vi "Timing Page.vi"(8 "error in (no error)":errorcluster, 11 "Node Ptr":T1 format="%.0x") -> (0 "error out":errorcluster)   [LabVIEW 2020, in "Engine Simulation Toolkit System Explorer.lvlib"]
uses:
  Engine Simulation Toolkit System Explorer.lvlib
  <vilib>/NI VeriStand/Custom Device API/Custom Device Item Ref.ctl
  Shared/Properties.vi
  <vilib>/NI VeriStand/Custom Device API/Get Item Property (Double).vi
  Shared/Constants and GUIDs.vi
  <vilib>/NI VeriStand/Custom Device API/Set Item Property (Double).vi
  <vilib>/NI VeriStand/Custom Device API/Custom Device API.lvlib
  Shared/Engine Simulation Toolkit Shared.lvlib
panel:
  in  "Stuck active\nlimit (ms)":dbl min=0.0 max=209.7152 step=0.0008
  in  "Header 2":cluster{"Section Name":string}={"Section Name"="Measurements"}
  in  "remove meas":bool
  in  "add meas":bool
  in  "remove windows":bool
  in  "add window":bool
  in  "windows listbox":i32[](listbox) caption="Window Definitions"
  in  "meas listbox":i32[](listbox) caption="Measurements"
  in  "Header":cluster{"Section Name":string}={"Section Name"="Measurement Windows"}
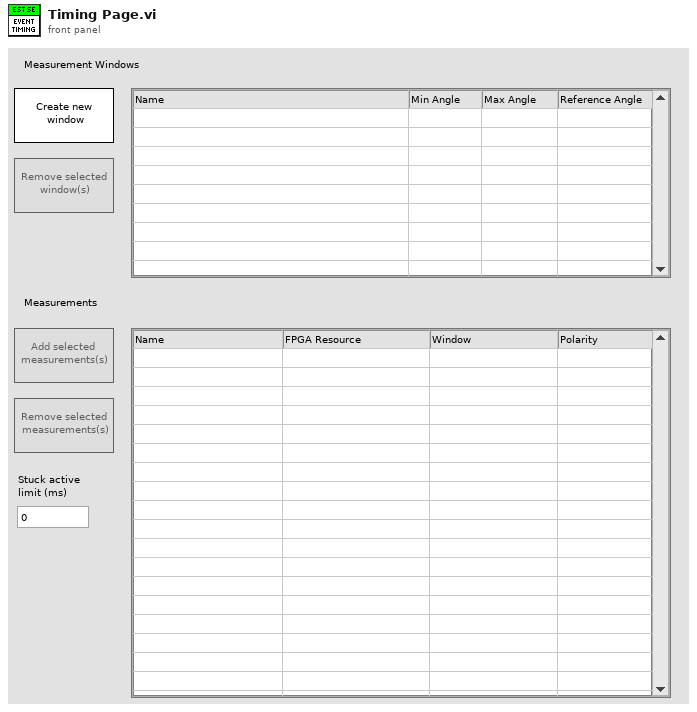
[diagram p1: front panel]
types:
  T1 = typedef "Custom Device API.lvlib/Custom Device Item Ref.ctl" = u64
  T2 = enum8{"Enabled", "Disabled", "Disabled and Grayed Out"}
  T3 = typedef "Engine Simulation Toolkit System Explorer.lvlib/Event Timing Window.ctl" = cluster{"Name":string, "Min":dbl, "Max":dbl, "Ref":dbl}
  T4 = typedef "Engine Simulation Toolkit System Explorer.lvlib/Event Timing Measurement.ctl" = cluster{"Name":string, "Bitfile name":string, "Window":string, "Polarity":T5}
  T5 = typedef "Engine Simulation Toolkit System Explorer.lvlib/Polarity.ctl" = enum16{"Active low", "Active high"}
  T6 = typedef "Custom Device API.lvlib/Custom Device Commands.ctl" = enum16{"Default", "Item renamed", "Shutdown", "Dynamic button pressed"}
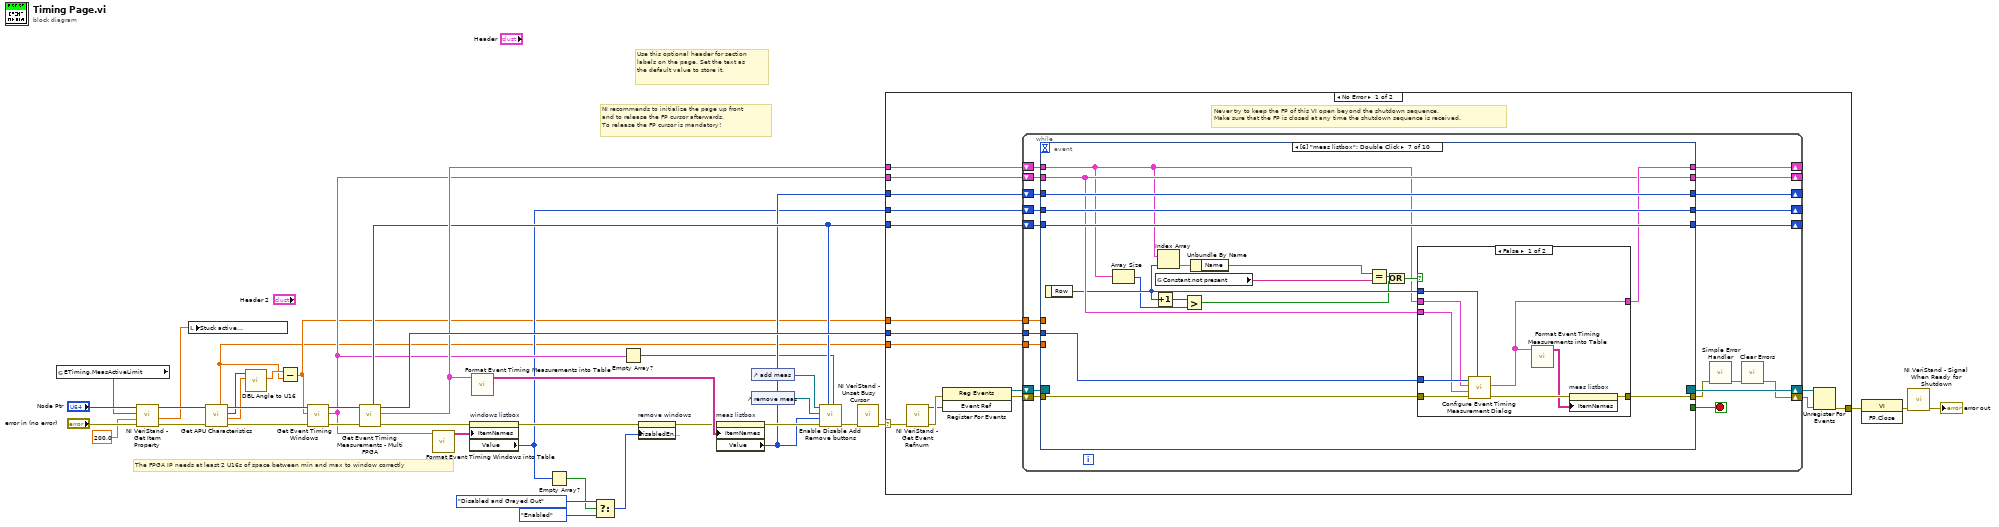
[diagram p0: block diagram]
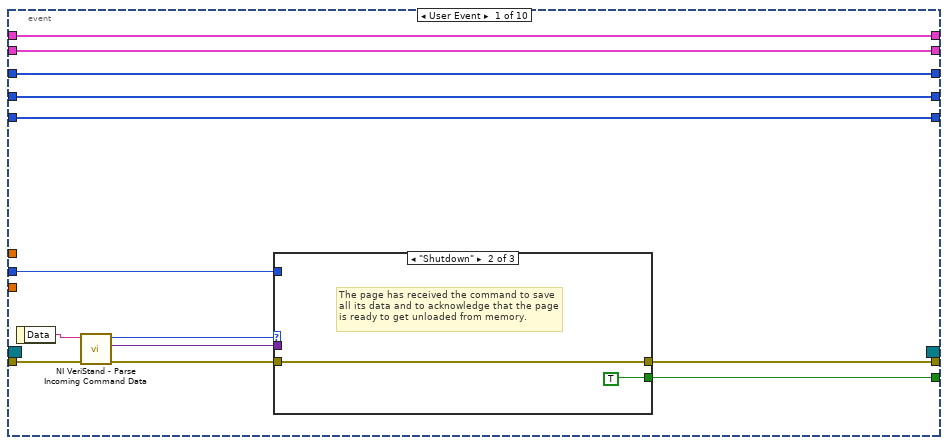
[diagram p2: hidden frame]
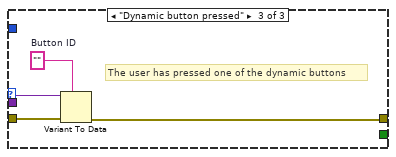
[diagram p4: hidden frame]
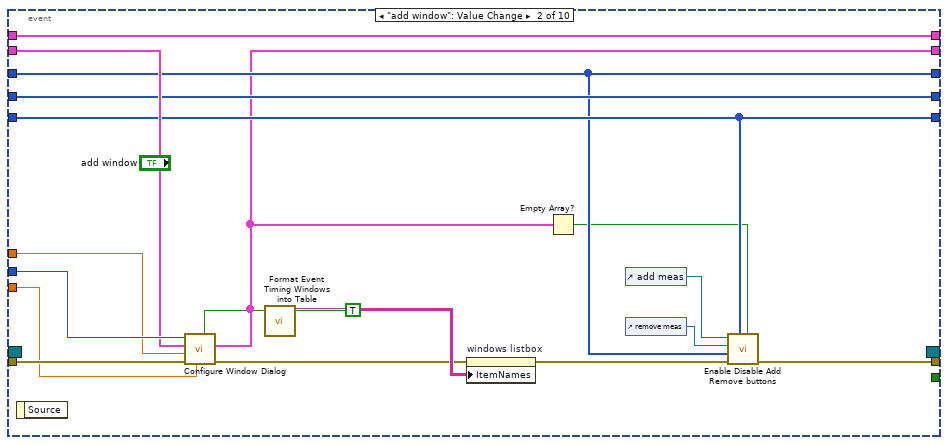
[diagram p5: hidden frame]
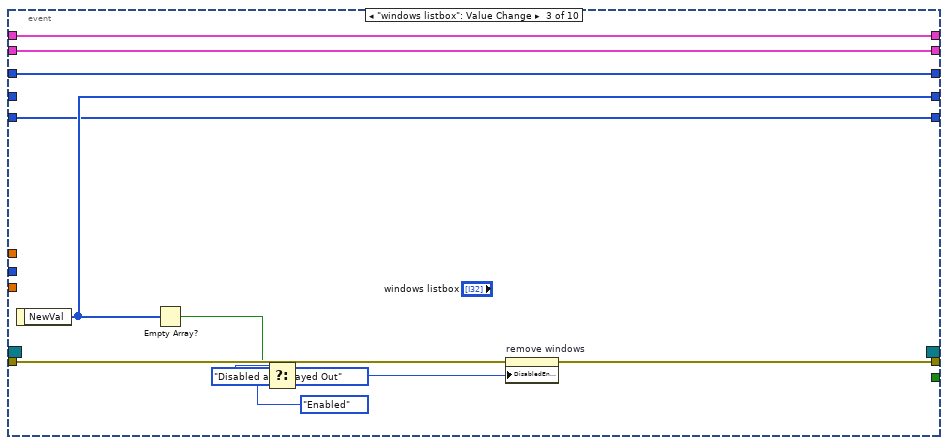
[diagram p6: hidden frame]
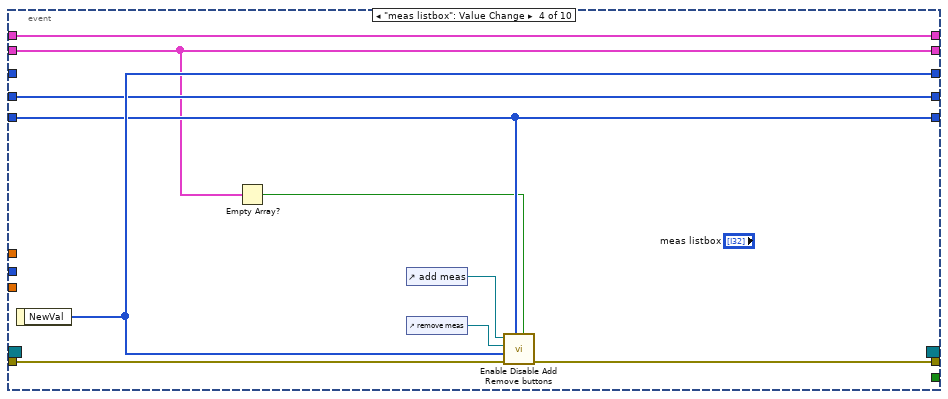
[diagram p7: hidden frame]
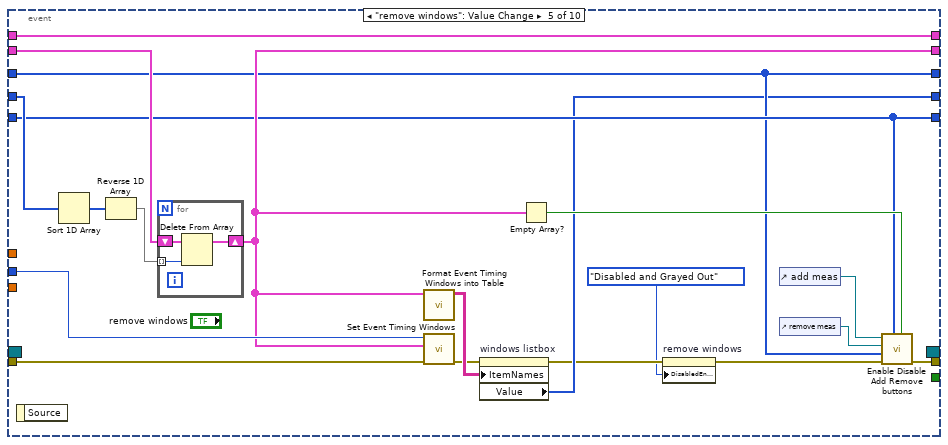
[diagram p8: hidden frame]
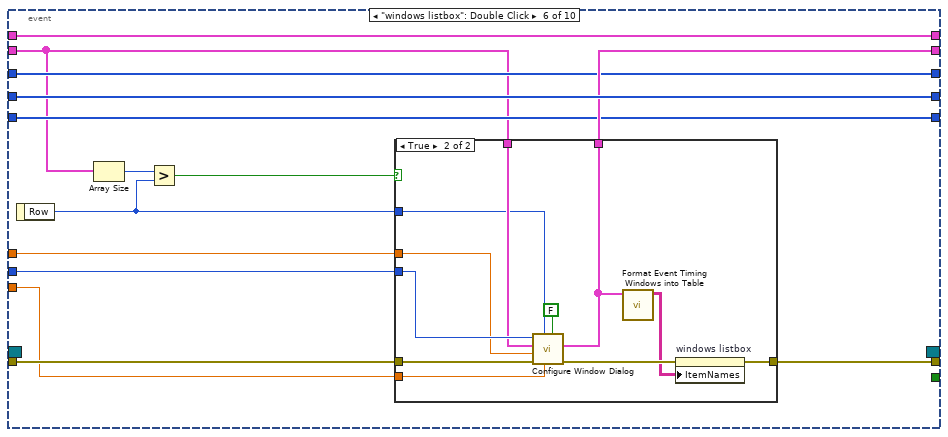
[diagram p9: hidden frame]
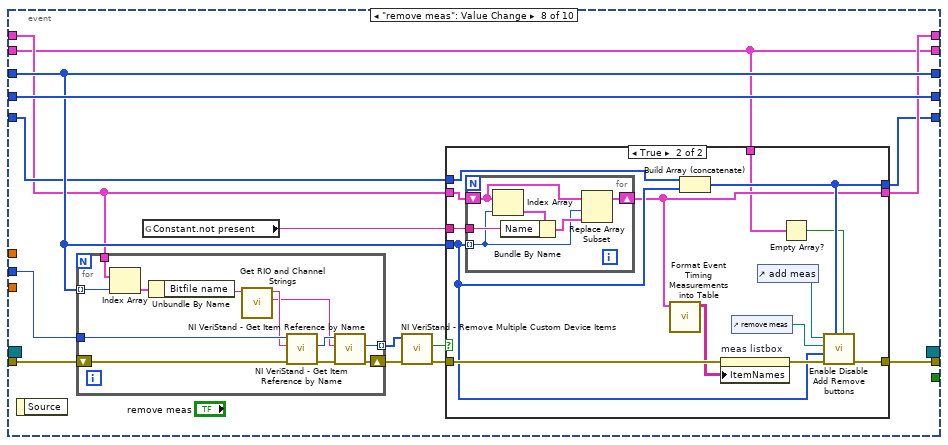
[diagram p12: hidden frame]
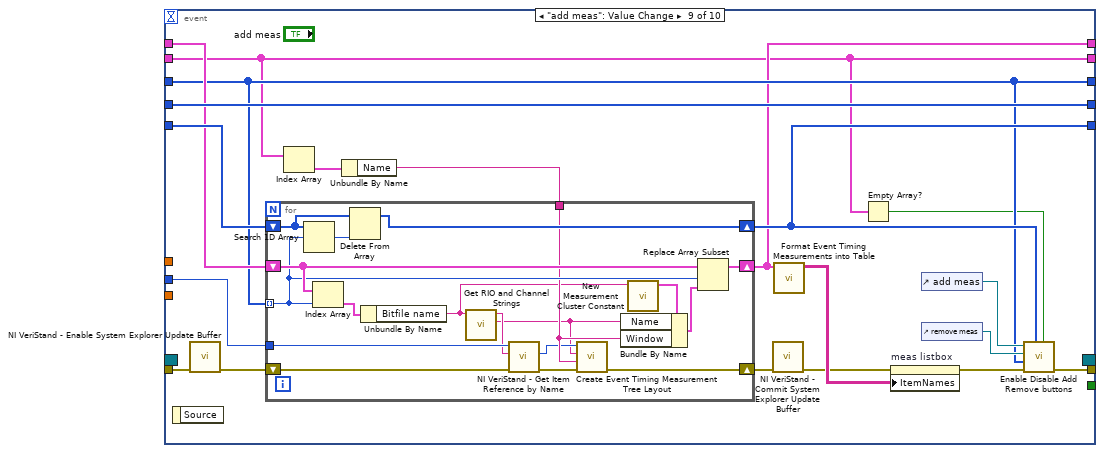
[diagram p14: hidden frame]
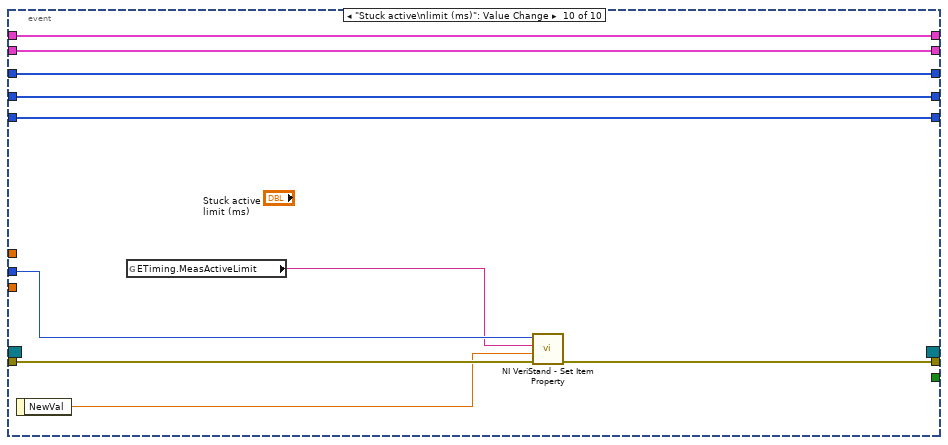
[diagram p15: hidden frame]
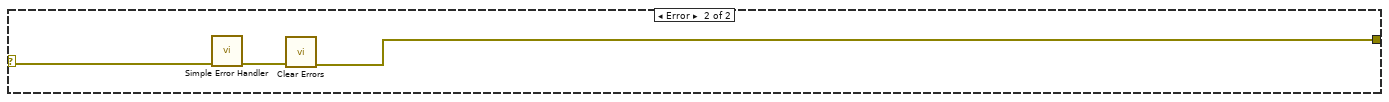
[diagram p16: hidden frame]
diagram:
  # "The FPGA IP needs at least 2 U16s of space between min and max to window correctly"
  # "Use this optional header for section labels on the page. Set the text as the default value to store it."
  # "NI recommends to initialize the page up front\nand to release the FP cursor afterwards.\nTo release the FP cursor is mandatory!"
  n1 = global read "Properties.vi" "ETiming.MeasActiveLimit"() -> (w7:string)
  n2 = call-poly <vilib>:"NI VeriStand - Get Item Property.vi"("error in (no error)"="error in (no error)", "Default Value"=200.0, "Property Name"=w7, "Item Ref in"="Node Ptr") -> ("error out"=w10:errorcluster, "Value"=w5:dbl, "Item Ref out"=w8:T1)  [unwired: 4 in, 1 out]
  n3 = local write "Stuck active\nlimit (ms)"(w5) -> ()
  n4 = call "Get APU Characteristics.vi"("error in (no error)"=w10, "Item Ref in"=w8) -> ("error out"=w35:errorcluster, "angle to u16 scale factor"=w31:dbl, "total angle span (degrees)"=w32:u16, "Item Ref out"=w34:T1, "degrees of one u16"=w1:dbl)  [unwired: 3 in, 2 out]
  n5 = call "DBL Angle to U16.vi"("angle to u16 scale factor"=w31, "Desired angle (degrees)"=w32) -> ("Actual angle (degrees)"=w33:dbl)  [unwired: 8 in, 1 out]
  n6 = Subtract(x=w33, y=w1) -> (x-y=w2:dbl)
  n7 = call "Get Event Timing Windows.vi"("error in (no error)"=w35, "Max engine angle"=w2, "Item Ref in"=w34) -> ("error out"=w28:errorcluster, "Windows"=w12:T3[], "Item Ref out"=w29:T1)  [unwired: 6 in]
  n8 = call "Get Event Timing Measurements - Multi FPGA.vi"("error in (no error)"=w28, "Item Ref in"=w29) -> ("error out"=w27:errorcluster, "measurements"=w24:T4[], "Item Ref out"=w26:T1, "not present indexes"=w14:i32[])  [unwired: 5 in, 1 out]
  n9 = call "Format Event Timing Windows into Table.vi"("Windows"=w12) -> ("Table"=w36:string[][])  [unwired: 10 in]
  n10 = property on="windows listbox" class="MCListbox (strict)"(error in=w27, "ItemNames"=w36) -> (error out=w23:errorcluster, "Value"=w4:i32[])  [unwired: 1 in, 1 out]
  n11 = call "Format Event Timing Measurements into Table.vi"("Measurements"=w24) -> ("Table"=w25:string[][])  [unwired: 10 in]
  n12 = Empty Array?(array=w4) -> (empty?=w3:bool)
  n13 = Select(t=T2."Disabled and Grayed Out" ("Disabled"), s=w3, f=T2."Enabled" ("Disabled")) -> (s? t:f=w19:T2)
  n14 = Empty Array?(array=w12) -> (empty?=w11:bool)
  n15 = property on="remove windows" class="Bool"(error in=w23, "DisabledEnum"=w19) -> (error out=w22:errorcluster)  [unwired: 1 in, 1 out]
  n16 = property on="meas listbox" class="MCListbox (strict)"(error in=w22, "ItemNames"=w25) -> (error out=w15:errorcluster, "Value"=w13:i32[])  [unwired: 1 in, 1 out]
  n17 = control-ref of="add meas"() -> (w17:refnum<vi>)
  n18 = control-ref of="remove meas"() -> (w18:refnum<vi>)
  n19 = call "Enable Disable Add Remove buttons.vi"("Force add disabled (F)"=w11, "not present item indexes"=w14, "error in (no error)"=w15, "selected items"=w13, "remove button"=w18, "add button"=w17) -> ("error out"=w16:errorcluster)  [unwired: 5 in]
  n20 = call <vilib>:"NI VeriStand - Unset Busy Cursor.vi"("error in (no error)"=w16) -> ("error out"=w37:errorcluster)  [unwired: 10 out]
  n21 = case shown="No Error" w37 {
    selector: w37 -> [w48 w315]
    tunnel: [w53 w313] -> w40
    tunnel: w26 -> [w49 _]
    tunnel: w12 -> [w47 _]
    tunnel: w2 -> [w46 _]
    tunnel: w1 -> [w45 _]
    tunnel: w24 -> [w44 _]
    tunnel: w14 -> [w43 _]
    tunnel: w4 -> [w42 _]
    tunnel: w13 -> [w41 _]
    frame No Error {
      # "Never try to keep the FP of this VI open beyond the shutdown sequence.\nMake sure that the FP is closed at any time the shutdown sequence is received."
      n22 = call <vilib>:"NI VeriStand - Get Event Refnum.vi"("error in (no error)"=w48) -> ("error out"=w56:errorcluster, "Event Ref"=w52:refnum<user-event>)  [unwired: 9 out]
      n23 = register-events(error in=w56, w52) -> (reference out=w50:refnum<event-registration>, error out=w51:errorcluster)  [unwired: 1 in]
      n24 = while {
        tunnel: w49 -> [w72]
        shift-right: [w69] -> w54
        shift-left: w51 -> [w75]
        shift-right: [w76] -> w55
        shift-left: w50 -> [w74]
        shift-right: [w67] -> _
        shift-left: w47 -> [w68]
        tunnel: w46 -> [w66]
        tunnel: w45 -> [w65]
        shift-right: [w64] -> _
        shift-left: w42 -> [w63]
        shift-right: [w58] -> _
        shift-left: w44 -> [w62]
        shift-right: [w61] -> _
        shift-left: w41 -> [w60]
        shift-right: [w57] -> _
        shift-left: w43 -> [w59]
        stop <- w73 stop-if-true
        n25 = event shown="[6] \"meas listbox\": Double Click" {
          selector: w74 -> [_ _ _ _ _ _ _ _ _ _]
          dyn-events: [_ _ _ _ _ _ _ _ _ _] -> w76
          timeout: _ -> [_ _ _ _ _ _ _ _ _ _]
          tunnel: w75 -> [w89 w114 w119 w134 w151 w172 w203 w223 w279 w312]
          tunnel: [w85 _ _ _ _ _ _ _ _ _] -> w73
          tunnel: [w84 w101 w124 w135 w143 w167 w200 w222 w283 w306] -> w71
          tunnel: w72 -> [w83 w113 _ _ w150 w171 w202 w221 w276 w304]
          tunnel: w68 -> [w81 w112 w125 w127 w155 w159 w196 w215 w266 w311]
          tunnel: [w81 w98 w125 w127 w142 w166 w196 w215 w266 w311] -> w67
          tunnel: w66 -> [_ w111 _ _ _ w170 _ _ _ _]
          tunnel: w65 -> [_ w109 _ _ _ w169 _ _ _ _]
          tunnel: [w80 w106 w123 w130 w139 w168 w201 w229 w284 w310] -> w64
          tunnel: w63 -> [w80 w106 _ w130 w154 w168 w201 w229 w284 w310]
          tunnel: w62 -> [w78 w105 w117 w128 w147 w163 w189 w218 w275 w308]
          tunnel: [w79 w99 w118 w131 w140 w165 w199 w220 w272 w309] -> w61
          tunnel: w60 -> [w79 w99 w118 _ w140 w165 w199 w220 w272 w309]
          tunnel: w59 -> [w77 w100 w116 w129 w141 w164 w198 w219 w277 w307]
          tunnel: [w78 w105 w117 w128 w147 w163 w197 w217 w271 w308] -> w58
          tunnel: [w77 w100 w116 w129 w141 w164 w198 w216 w273 w307] -> w57
          event User Event {
            n26 = event-data() -> ("Data"=w88:string)  [unwired: 1 out]
            n27 = call <vilib>:"NI VeriStand - Parse Incoming Command Data.vi"("error in (no error)"=w89, "Incoming data"=w88) -> ("error out"=w87:errorcluster, "Outgoing data"=w82:variant, "Action"=w86:T6)  [unwired: 7 out]
            n28 = case shown="\"Shutdown\"" w86 {
              tunnel: w87 -> [w90 w91 w96]
              tunnel: [_ TRUE _] -> w85
              tunnel: [w90 w91 w93] -> w84
              tunnel: w83 -> [_ _ _]
              tunnel: w82 -> [_ _ w95]
              frame "Default", Default {
              }
              frame "Shutdown" {
                # "The page has received the command to save all its data and to acknowledge that the page is ready to get unloaded from memory."
              }
              frame "Dynamic button pressed" {
                w94 = ""  # Button ID
                # "The user has pressed one of the dynamic buttons"
                n29 = Variant To Data(error in=w96, type=w94, Variant=w95) -> (error out=w93:errorcluster)  [unwired: 1 out]
              }
            }
          }
          event "add window": Value Change {
            n30 = event-data() -> ()  [unwired: 2 out]
            n31 = call "Configure Window Dialog.vi"("New"=TRUE, "degrees of one u16"=w109, "error in (no error)"=w114, "Max engine angle"=w111, "windows in"=w112, "Item Ref in"=w113) -> ("error out"=w107:errorcluster, "windows out"=w98:T3[])  [unwired: 3 in, 1 out]
            n32 = call "Format Event Timing Windows into Table.vi"("Windows"=w98) -> ("Table"=w108:string[][])  [unwired: 10 in]
            n33 = property on="windows listbox" class="MCListbox (strict)"(error in=w107, "ItemNames"=w108) -> (error out=w102:errorcluster)  [unwired: 1 in, 1 out]
            n34 = Empty Array?(array=w98) -> (empty?=w97:bool)
            n35 = control-ref of="add meas"() -> (w104:refnum<vi>)
            n36 = control-ref of="remove meas"() -> (w103:refnum<vi>)
            n37 = call "Enable Disable Add Remove buttons.vi"("Force add disabled (F)"=w97, "not present item indexes"=w100, "error in (no error)"=w102, "selected items"=w99, "remove button"=w103, "add button"=w104) -> ("error out"=w101:errorcluster)  [unwired: 5 in]
          }
          event "windows listbox": Value Change {
            n38 = event-data() -> ("NewVal"=w123:i32[])  [unwired: 1 out]
            n39 = Empty Array?(array=w123) -> (empty?=w115:bool)
            n40 = Select(t=T2."Disabled and Grayed Out" ("Disabled"), s=w115, f=T2."Enabled" ("Disabled")) -> (s? t:f=w120:T2)
            n41 = property on="remove windows" class="Bool"(error in=w119, "DisabledEnum"=w120) -> (error out=w124:errorcluster)  [unwired: 1 in, 1 out]
          }
          event "meas listbox": Value Change {
            n42 = event-data() -> ("NewVal"=w131:i32[])  [unwired: 1 out]
            n43 = Empty Array?(array=w127) -> (empty?=w126:bool)
            n44 = control-ref of="add meas"() -> (w133:refnum<vi>)
            n45 = control-ref of="remove meas"() -> (w132:refnum<vi>)
            n46 = call "Enable Disable Add Remove buttons.vi"("Force add disabled (F)"=w126, "not present item indexes"=w129, "error in (no error)"=w134, "selected items"=w131, "remove button"=w132, "add button"=w133) -> ("error out"=w135:errorcluster)  [unwired: 5 in]
          }
          event "remove windows": Value Change {
            n47 = event-data() -> ()  [unwired: 2 out]
            n48 = Sort 1D Array(array=w154) -> (sorted array=w153:i32[])
            n49 = Reverse 1D Array(array=w153) -> (reversed array=w152:i32[])
            n50 = for {
              tunnel: w152 -> [w157] mode=indexing
              shift-right: [w156] -> w142
              shift-left: w155 -> [w158]
              n51 = Delete From Array(array=w158, index=w157) -> (array with subset deleted=w156:T3[])  [unwired: 1 in, 1 out]
            }
            n52 = call "Format Event Timing Windows into Table.vi"("Windows"=w142) -> ("Table"=w149:string[][])  [unwired: 10 in]
            n53 = call "Set Event Timing Windows.vi"("error in (no error)"=w151, "Windows"=w142, "Item Ref in"=w150) -> ("error out"=w148:errorcluster)  [unwired: 7 in, 1 out]
            n54 = property on="windows listbox" class="MCListbox (strict)"(error in=w148, "ItemNames"=w149) -> (error out=w138:errorcluster, "Value"=w139:i32[])  [unwired: 1 in, 1 out]
            n55 = Empty Array?(array=w142) -> (empty?=w144:bool)
            n56 = property on="remove windows" class="Bool"(error in=w138, "DisabledEnum"=T2."Disabled and Grayed Out" ("Disabled")) -> (error out=w137:errorcluster)  [unwired: 1 in, 1 out]
            n57 = control-ref of="add meas"() -> (w146:refnum<vi>)
            n58 = control-ref of="remove meas"() -> (w145:refnum<vi>)
            n59 = call "Enable Disable Add Remove buttons.vi"("Force add disabled (F)"=w144, "not present item indexes"=w141, "error in (no error)"=w137, "selected items"=w140, "remove button"=w145, "add button"=w146) -> ("error out"=w143:errorcluster)  [unwired: 5 in]
          }
          event "windows listbox": Double Click {
            n60 = event-data() -> ("Row"=w160:i32)  [unwired: 1 out]
            n61 = Array Size(array=w159) -> (size(s)=w161:i32)
            n62 = Greater?(x=w161, y=w160) -> (0:w162:bool)
            n63 = case shown="True" w162 {
              tunnel: w172 -> [w173 w185]
              tunnel: w171 -> [_ w184]
              tunnel: w159 -> [w174 w183]
              tunnel: w170 -> [_ w182]
              tunnel: w169 -> [_ w180]
              tunnel: w160 -> [_ w179]
              tunnel: [w173 w177] -> w167
              tunnel: [w174 w176] -> w166
              frame False {
              }
              frame True {
                n64 = call "Configure Window Dialog.vi"("New"=FALSE, "degrees of one u16"=w180, "Window to be edited"=w179, "error in (no error)"=w185, "Max engine angle"=w182, "windows in"=w183, "Item Ref in"=w184) -> ("error out"=w178:errorcluster, "windows out"=w176:T3[])  [unwired: 2 in, 1 out]
                n65 = call "Format Event Timing Windows into Table.vi"("Windows"=w176) -> ("Table"=w175:string[][])  [unwired: 10 in]
                n66 = property on="windows listbox" class="MCListbox (strict)"(error in=w178, "ItemNames"=w175) -> (error out=w177:errorcluster)  [unwired: 1 in, 1 out]
              }
            }
          }
          event "meas listbox": Double Click {
            n67 = event-data() -> ("Row"=w190:i32)  [unwired: 1 out]
            n68 = Array Size(array=w189) -> (size(s)=w188:i32)
            n69 = Increment(x=w190) -> (x+1=w186:i32)
            n70 = global read "Constants and GUIDs.vi" "Constant.not present"() -> (w194:string)
            n71 = Index Array(array=w189, index=w190) -> (element=w195:T4)
            n72 = Greater?(x=w186, y=w188) -> (0:w187:bool)
            n73 = Unbundle By Name(w195) -> ("Name"=w193:string)
            n74 = Equal?(x=w193, y=w194) -> (x = y?=w192:bool)
            n75 = Or(x=w192, y=w187) -> (x .or. y?=w191:bool)
            n76 = case shown="False" w191 {
              tunnel: w203 -> [w212 w213]
              tunnel: w202 -> [w211 _]
              tunnel: [w209 w213] -> w200
              tunnel: [w207 w214] -> w197
              tunnel: w196 -> [w206 _]
              tunnel: w189 -> [w205 w214]
              tunnel: w190 -> [w204 _]
              frame False {
                n77 = call "Configure Event Timing Measurement Dialog.vi"("measurement to be edited"=w204, "error in (no error)"=w212, "windows"=w206, "measurements in"=w205, "Item Ref in"=w211) -> ("error out"=w210:errorcluster, "measurements out"=w207:T4[])  [unwired: 4 in, 1 out]
                n78 = call "Format Event Timing Measurements into Table.vi"("Measurements"=w207) -> ("Table"=w208:string[][])  [unwired: 10 in]
                n79 = property on="meas listbox" class="MCListbox (strict)"(error in=w210, "ItemNames"=w208) -> (error out=w209:errorcluster)  [unwired: 1 in, 1 out]
              }
              frame True {
              }
            }
          }
          event "remove meas": Value Change {
            n80 = event-data() -> ()  [unwired: 2 out]
            n81 = for {
              tunnel: w220 -> [w261] mode=indexing
              tunnel: w218 -> [w262]
              tunnel: w221 -> [w257]
              tunnel: [w263] -> w225 mode=indexing
              shift-right: [w264] -> w224
              shift-left: w223 -> [w258]
              n82 = Index Array(array=w262, index=w261) -> (element=w260:T4)
              n83 = Unbundle By Name(w260) -> ("Bitfile name"=w255:string)
              n84 = call "Get RIO and Channel Strings.vi"("rio/channel"=w255) -> ("channel"=w253:string, "rio"=w254:string)  [unwired: 9 in]
              n85 = call <vilib>:"NI VeriStand - Get Item Reference by Name.vi"("error in (no error)"=w258, "Item Name"=w254, "Parent Ref in"=w257) -> ("error out"=w259:errorcluster, "Item Ref"=w256:T1)  [unwired: 5 in, 2 out]
              n86 = call <vilib>:"NI VeriStand - Get Item Reference by Name.vi"("error in (no error)"=w259, "Item Name"=w253, "Parent Ref in"=w256) -> ("error out"=w264:errorcluster, "Item Ref"=w263:T1)  [unwired: 5 in, 2 out]
            }
            n87 = global read "Constants and GUIDs.vi" "Constant.not present"() -> (w228:string)
            n88 = call <vilib>:"NI VeriStand - Remove Multiple Custom Device Items.vi"("error in (no error)"=w224, "Item Refs in"=w225) -> ("error out"=w226:errorcluster, "Deleted?"=w227:bool)  [unwired: 8 in]
            n89 = case shown="True" w227 {
              tunnel: [w231 w245] -> w222
              tunnel: w226 -> [w231 w244]
              tunnel: w220 -> [_ w240]
              tunnel: w218 -> [w232 w243]
              tunnel: w228 -> [_ w242]
              tunnel: [w232 w236] -> w217
              tunnel: w219 -> [w230 w241]
              tunnel: [w230 w239] -> w216
              tunnel: w215 -> [_ w234]
              frame False {
              }
              frame True {
                n90 = for {
                  tunnel: w240 -> [w247] mode=indexing
                  shift-right: [w249] -> w236
                  shift-left: w243 -> [w250]
                  tunnel: w242 -> [w251]
                  n91 = Index Array(array=w250, index=w247) -> (element=w252:T4)
                  n92 = Bundle By Name(cluster=w252, "Name"=w251) -> (w248:T4)
                  n93 = Replace Array Subset(array=w250, new element=w248, index=w247) -> (w249:T4[])
                }
                n94 = call "Format Event Timing Measurements into Table.vi"("Measurements"=w236) -> ("Table"=w235:string[][])  [unwired: 10 in]
                n95 = Build Array (concatenate)(w241, w240) -> (w239:i32[])
                n96 = property on="meas listbox" class="MCListbox (strict)"(error in=w244, "ItemNames"=w235) -> (error out=w246:errorcluster)  [unwired: 1 in, 1 out]
                n97 = control-ref of="remove meas"() -> (w237:refnum<vi>)
                n98 = control-ref of="add meas"() -> (w238:refnum<vi>)
                n99 = Empty Array?(array=w234) -> (empty?=w233:bool)
                n100 = call "Enable Disable Add Remove buttons.vi"("Force add disabled (F)"=w233, "not present item indexes"=w239, "error in (no error)"=w246, "selected items"=w240, "remove button"=w237, "add button"=w238) -> ("error out"=w245:errorcluster)  [unwired: 5 in]
              }
            }
          }
          event "add meas": Value Change {
            n101 = event-data() -> ()  [unwired: 2 out]
            n102 = call <vilib>:"NI VeriStand - Enable System Explorer Update Buffer.vi"("error in (no error)"=w279) -> ("error out"=w270:errorcluster)  [unwired: 10 in]
            n103 = Index Array(array=w266) -> (element=w268:T3)  [unwired: 1 in]
            n104 = Unbundle By Name(w268) -> ("Name"=w267:string)
            n105 = for {
              tunnel: w276 -> [w288]
              shift-right: [w302] -> w278
              shift-left: w270 -> [w289]
              tunnel: w272 -> [w299] mode=indexing
              shift-right: [w300] -> w271
              shift-left: w275 -> [w301]
              shift-right: [w296] -> w273
              shift-left: w277 -> [w298]
              tunnel: w267 -> [w292]
              n106 = Search 1D Array(1D array=w298, element=w299) -> (index of element=w297:i32)  [unwired: 1 in]
              n107 = Index Array(array=w301, index=w299) -> (element=w295:T4)
              n108 = Delete From Array(array=w298, index=w297) -> (array with subset deleted=w296:i32[])  [unwired: 1 in, 1 out]
              n109 = Unbundle By Name(w295) -> ("Bitfile name"=w291:string)
              n110 = call "Get RIO and Channel Strings.vi"("rio/channel"=w291) -> ("channel"=w285:string, "rio"=w286:string)  [unwired: 9 in]
              n111 = call <vilib>:"NI VeriStand - Get Item Reference by Name.vi"("error in (no error)"=w289, "Item Name"=w286, "Parent Ref in"=w288) -> ("error out"=w290:errorcluster, "Item Ref"=w287:T1)  [unwired: 5 in, 2 out]
              n112 = call "Create Event Timing Measurement Tree Layout.vi"("error in (no error)"=w290, "window"=w292, "measurement name"=w285, "Section Ptr"=w287) -> ("error out"=w302:errorcluster)  [unwired: 6 in, 1 out]
              n113 = call "New Measurement Cluster Constant.vi"("Bitfile name"=w291) -> ("Measurement"=w293:T4)  [unwired: 10 in]
              n114 = Bundle By Name(cluster=w293, "Name"=w285, "Window"=w292) -> (w294:T4)
              n115 = Replace Array Subset(array=w301, new element=w294, index=w299) -> (w300:T4[])
            }
            n116 = call <vilib>:"NI VeriStand - Commit System Explorer Update Buffer.vi"("error in (no error)"=w278) -> ("error out"=w269:errorcluster)  [unwired: 10 in]
            n117 = call "Format Event Timing Measurements into Table.vi"("Measurements"=w271) -> ("Table"=w274:string[][])  [unwired: 10 in]
            n118 = Empty Array?(array=w266) -> (empty?=w265:bool)
            n119 = property on="meas listbox" class="MCListbox (strict)"(error in=w269, "ItemNames"=w274) -> (error out=w282:errorcluster)  [unwired: 1 in, 1 out]
            n120 = control-ref of="add meas"() -> (w281:refnum<vi>)
            n121 = control-ref of="remove meas"() -> (w280:refnum<vi>)
            n122 = call "Enable Disable Add Remove buttons.vi"("Force add disabled (F)"=w265, "not present item indexes"=w273, "error in (no error)"=w282, "selected items"=w272, "remove button"=w280, "add button"=w281) -> ("error out"=w283:errorcluster)  [unwired: 5 in]
          }
          event "Stuck active\nlimit (ms)": Value Change {
            n123 = event-data() -> ("NewVal"=w305:dbl)  [unwired: 1 out]
            n124 = global read "Properties.vi" "ETiming.MeasActiveLimit"() -> (w303:string)
            n125 = call-poly <vilib>:"NI VeriStand - Set Item Property.vi"("error in (no error)"=w312, "Value"=w305, "Property Name"=w303, "Item Ref in"=w304) -> ("error out"=w306:errorcluster)  [unwired: 5 in, 2 out]
          }
        }
        n126 = call <vilib>:"Simple Error Handler.vi"("error in (no error)"=w71) -> ("error out"=w70:errorcluster)  [unwired: 1 in, 7 out]
        n127 = call <vilib>:"Clear Errors.vi"("error in (no error)"=w70) -> ("error out"=w69:errorcluster)  [unwired: 1 in, 5 out]
      }
      n128 = Unregister For Events(event registration refnum=w55, error in=w54) -> (error out=w53:errorcluster)
    }
    frame Error {
      n129 = call <vilib>:"Simple Error Handler.vi"("error in (no error)"=w315) -> ("error out"=w314:errorcluster)  [unwired: 1 in, 7 out]
      n130 = call <vilib>:"Clear Errors.vi"("error in (no error)"=w314) -> ("error out"=w313:errorcluster)  [unwired: 1 in, 5 out]
    }
  }
  n131 = invoke class="VI" method="FP.Close"(error in=w40) -> (error out=w39:errorcluster)  [unwired: 2 in, 2 out]
  n132 = call <vilib>:"NI VeriStand - Signal When Ready for Shutdown.vi"("error in (no error)"=w39) -> ("error out"=→"error out":errorcluster)  [unwired: 10 out]
